vi "surface analysis.vi"() -> ()   [LabVIEW 2018]
uses:
  Program Files (x86)/National Instruments/LabVIEW 2018/examples/Connectivity/Python/support/PythonVersionsEnum.ctl
  PythonConfigGlobal.vi
panel:
  in  "탭 컨트롤":T1(tab)
  in  "python version":T2=enum."3.6"
  in  "auto select":bool=TRUE
  in  "p value 기준":dbl=0.30000000000000004 format="%#_13g"
  in  "min max":dbl[][](array[numeric])=[[4.0, 10.0], [50.0, 150.0], [0.5, 1.5]]
  in  "요인":string[](array[string])=["x1", "x2", "x3"]
  in  "비용목표":string[](array[string])=["y1"]
  in  "min":dbl[](array[numeric])
  in  "max":dbl[](array[numeric])
  out "최소화":bool[](array[boolean])
  out "CCD":dbl[][](array[numeric])=[[0.0, 1.0, 1.0], [-1.0, 0.0, -1.0], [1.0, -1.0, 0.0], [0.0, -1.0, 1.0], [0.0, 1.0, -1.0], [1.0, 1.0, 0.0], [0.0, 0.0, 0.0], [1.0, 0.0, 1.0], [0.0, 0.0, 0.0], [-1.0, -1.0, 0.0], [0.0, 0.0, 0.0], [-1.0, 0.0, 1.0], [1.0, 0.0, -1.0], [-1.0, 1.0, 0.0], [0.0, -1.0, -1.0]]
  out "요인 인디케이터":string[](array[string])=["x1", "x2", "x3"]
  out "결과":dbl[][](array[numeric])=[[-7664.4331863081525], [-4981.045086062967], [-2202.4239328817716], [-2350.3061672537383], [-7545.941821358417], [-7491.916698113938], [-4936.328310660356], [-4903.296353902461], [-4933.199416714428], [-2395.9779440706893], [-4933.81874642875], [-5116.35595558602], [-4793.002202085561], [-7680.887360331216], [-2246.212821164353]]
  out "비용 인디케이터":string[](array[string])=["y1"]
  out "시뮬레이션 인디케이터":string="시뮬레이션 횟수15/15\r\n인자 1 : 7.000000\r\n인자 2 : 50.000000\r\n인자 3 : 0.500000\r\n"
  in  "반복횟수":i32
  in  "정지":bool
  out "coef":dbl[](array[numeric])=[0.010139481576470908, 0.006600481306352523, 5.6726376890264e-10, 0.37234347257286826, 0.5641016129600653, 0.2140399578846797, 0.038152856088325596, 0.782518427242462, 0.17271126837436535, 0.40212171688452725]
  out "sumary":string="                            OLS Regression Results                            \n==============================================================================\nDep. Variable:                      y   R-squared:                       1.000\nModel:                            OLS   Adj. R-squared:                  1.000\nMethod:                 Least Squares   F-statistic:                 1.009e+05\nDate:                Sun, 20 Jan 2019   Prob (F-statistic):           1.32e-12\nTime:                        19:19:53   Log-Likelihood:                -43.985\nNo. Observations:                  15   AIC:                             108.0\nDf Residuals:                       5   BIC:                             115.0\nDf Model:                           9                                         \nCovariance Type:            nonrobust                                         \n==============================================================================\n                 coef    std err          t      P>|t|      [0.025      0.975]\n------------------------------------------------------------------------------\nconst        177.6892     44.222      4.018      0.010      64.013     291.365\nx1            33.1765      7.428      4.467      0.007      14.083      52.270\nx2           -52.3071      0.411   -127.305      0.000     -53.363     -51.251\nx3           -40.2432     41.088     -0.979      0.372    -145.863      65.377\nx4            -0.2808      0.455     -0.617      0.564      -1.450       0.889\nx5            -0.0023      0.002     -1.423      0.214      -0.007       0.002\nx6           -45.7962     16.377     -2.796      0.038     -87.893      -3.699\nx7            -0.0076      0.026     -0.291      0.783      -0.075       0.060\nx8             4.1695      2.622      1.590      0.173      -2.571      10.910\nx9            -0.1440      0.157     -0.915      0.402      -0.548       0.260\n==============================================================================\nOmnibus:                        0.092   Durbin-Watson:                   2.815\nProb(Omnibus):                  0.955   Jarque-Bera (JB):                0.320\nSkew:                          -0.003   Prob(JB):                        0.852\nKurtosis:                       2.284   Cond. No.                     3.73e+05\n==============================================================================\n\nWarnings:\n[1] Standard Errors assume that the covariance matrix of the errors is correctly specified.\n[2] The condition number is large, 3.73e+05. This might indicate that there are\nstrong multicollinearity or other numerical problems."
  out "name sort":string[](array[string])=["const", "x1 : x1", "x2 : x2", "x3 : x3", "x4 : x1^2", "x5 : x2^2", "x6 : x3^2", "x7 : x1*x2", "x8 : x1*x3", "x9 : x2*x3"]
  out "pValue sort":dbl[](array[numeric])=[0.010139481576470908, 0.006600481306352523, 5.6726376890264e-10, 0.37234347257286826, 0.5641016129600653, 0.2140399578846797, 0.038152856088325596, 0.782518427242462, 0.17271126837436535, 0.40212171688452725]
  in  "select":bool[](array[boolean])=[TRUE, TRUE, TRUE, TRUE, TRUE, TRUE, FALSE, FALSE, FALSE, FALSE]
  in  "선택완료":bool
  # "AUTO\nSELECT"
  # "1 2 3"
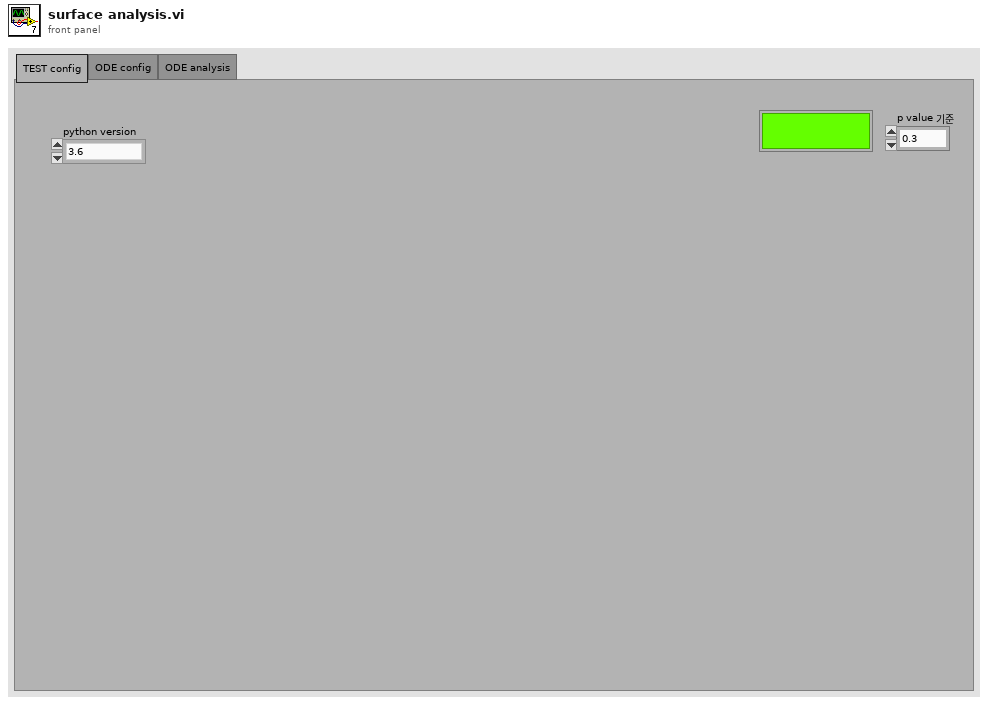
[diagram p1: front panel]
types:
  T1 = enum32{"TEST config", "ODE config", "ODE analysis"}
  T2 = typedef "PythonVersionsEnum.ctl" = enum16{"2.7", "3.6"}
  T3 = cluster{"session out":refnum<k35>, "appended path":path}
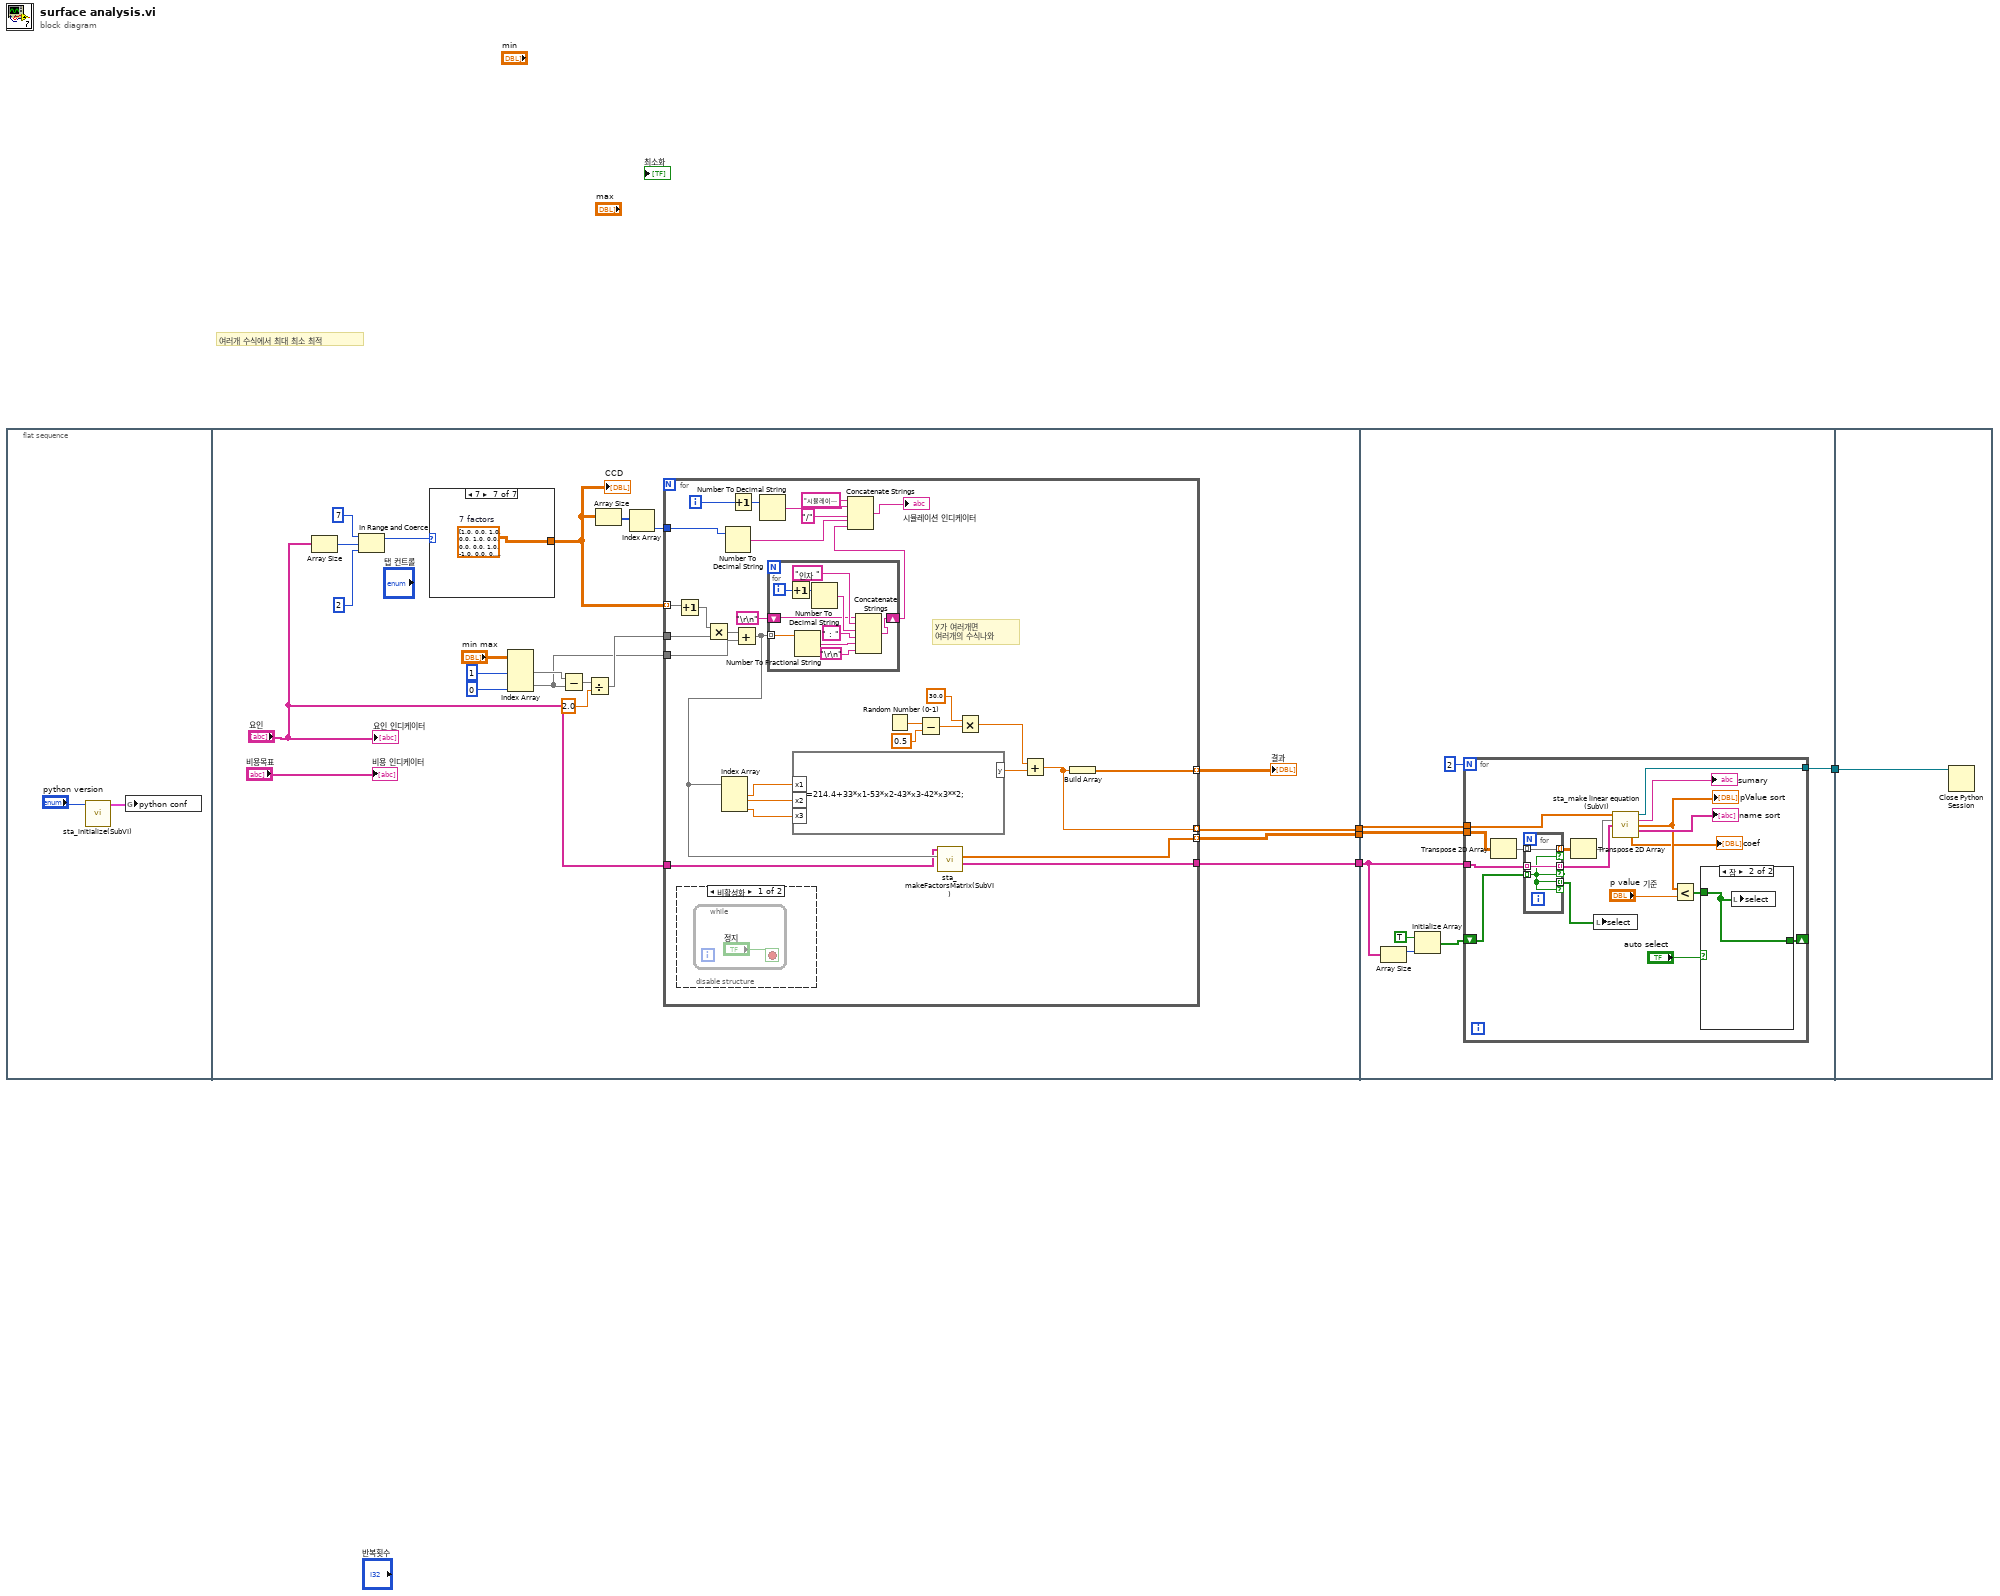
[diagram p0: block diagram]
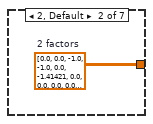
[diagram p4: hidden frame]
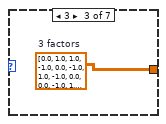
[diagram p5: hidden frame]
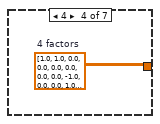
[diagram p6: hidden frame]
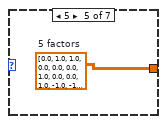
[diagram p7: hidden frame]
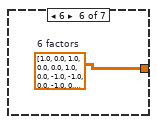
[diagram p8: hidden frame]
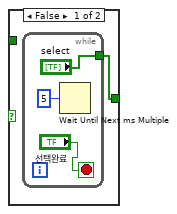
[diagram p9: hidden frame]
diagram:
  # "여러개 수식에서 최대 최소 최적"
  n1 = flat-sequence {
    tunnel: [w10] -> w4
    tunnel: [w9] -> w3
    tunnel: [w7] -> w1
    tunnel: w4 -> [w81]
    tunnel: w3 -> [w82]
    tunnel: [w80] -> w2
    tunnel: w1 -> [w77]
    tunnel: w2 -> [w109]
    frame #0 {
      n2 = call "sta_initialize(SubVI).vi"("python version"="python version") -> ("클러스터"=w5:T3)  [unwired: 10 in]
      n3 = global write "PythonConfigGlobal.vi" "python conf"(w5) -> ()
    }
    frame #1 {
      n4 = Array Size(array="요인") -> (size(s)=w26:i32)
      n5 = In Range and Coerce(upper limit=7 ("상위 리미트"), x=w26, lower limit=2 ("하위 리미트")) -> (coerced(x)=w23:i32)  [unwired: 1 out]
      n6 = case shown="7" w23 {
        tunnel: [_ w69 w70 w71 w72 w73 w74] -> w22
        frame 1 {
          # "황금비 추가"
        }
        frame 2, Default {
          w69 = dbl[][] [[0.0, 0.0], [-1.0, -1.0], [0.0, -1.41421], [0.0, 0.0], [0.0, 0.0], [1.41421, 0.0], [-1.0, 1.0], [-1.41421, 0.0], [0.0, 1.41421], [1.0, 1.0], [1.0, -1.0], [0.0, 0.0], [0.0, 0.0]]  # 2 factors
        }
        frame 3 {
          w70 = dbl[][] [[0.0, 1.0, 1.0], [-1.0, 0.0, -1.0], [1.0, -1.0, 0.0], [0.0, -1.0, 1.0], [0.0, 1.0, -1.0], [1.0, 1.0, 0.0], [0.0, 0.0, 0.0], [1.0, 0.0, 1.0], [0.0, 0.0, 0.0], [-1.0, -1.0, 0.0], [0.0, 0.0, 0.0], [-1.0, 0.0, 1.0], [1.0, 0.0, -1.0], [-1.0, 1.0, 0.0], [0.0, -1.0, -1.0]]  # 3 factors
        }
        frame 4 {
          w71 = dbl[][] [[1.0, 1.0, 0.0, 0.0], [0.0, 0.0, 0.0, 0.0], [-1.0, 0.0, 0.0, 1.0], [-1.0, -1.0, 0.0, 0.0], [0.0, 1.0, 1.0, 0.0], [-1.0, 0.0, 0.0, -1.0], [0.0, 0.0, 1.0, 1.0], [0.0, -1.0, -1.0, 0.0], [1.0, 0.0, -1.0, 0.0], [0.0, -1.0, 1.0, 0.0], [1.0, -1.0, 0.0, 0.0], [0.0, -1.0, 0.0, 1.0], [-1.0, 0.0, -1.0, 0.0], [0.0, 0.0, 0.0, 0.0], [1.0, 0.0, 0.0, -1.0], [1.0, 0.0, 0.0, 1.0], [0.0, -1.0, 0.0, -1.0], [0.0, 1.0, 0.0, 1.0], [0.0, 1.0, -1.0, 0.0], [-1.0, 0.0, 1.0, 0.0], [0.0, 0.0, 1.0, -1.0], [0.0, 0.0, -1.0, -1.0], [1.0, 0.0, 1.0, 0.0], [0.0, 0.0, 0.0, 0.0], [0.0, 1.0, 0.0, -1.0], [-1.0, 1.0, 0.0, 0.0], [0.0, 0.0, -1.0, 1.0]]  # 4 factors
        }
        frame 5 {
          w72 = dbl[][] [[0.0, 1.0, 1.0, 0.0, 0.0], [0.0, 1.0, 0.0, 0.0, 1.0], [-1.0, -1.0, 0.0, 0.0, 0.0], [0.0, 1.0, -1.0, 0.0, 0.0], [0.0, 0.0, 0.0, 0.0, 0.0], [0.0, 0.0, 0.0, 1.0, 1.0], [1.0, 1.0, 0.0, 0.0, 0.0], [0.0, 1.0, 0.0, 1.0, 0.0], [-1.0, 0.0, 1.0, 0.0, 0.0], [1.0, 0.0, 0.0, -1.0, 0.0], [0.0, 1.0, 0.0, 0.0, -1.0], [0.0, 0.0, 1.0, -1.0, 0.0], [0.0, 0.0, 0.0, 0.0, 0.0], [-1.0, 0.0, 0.0, -1.0, 0.0], [-1.0, 0.0, 0.0, 1.0, 0.0], [0.0, -1.0, 0.0, 1.0, 0.0], [0.0, 1.0, 0.0, -1.0, 0.0], [-1.0, 0.0, 0.0, 0.0, -1.0], [0.0, 0.0, 1.0, 0.0, -1.0], [0.0, 0.0, 0.0, 0.0, 0.0], [1.0, 0.0, 0.0, 0.0, 1.0], [1.0, -1.0, 0.0, 0.0, 0.0], [0.0, 0.0, 0.0, 1.0, -1.0], [0.0, 0.0, -1.0, 0.0, -1.0], [-1.0, 1.0, 0.0, 0.0, 0.0], [0.0, 0.0, 0.0, 0.0, 0.0], [0.0, 0.0, -1.0, -1.0, 0.0], [1.0, 0.0, -1.0, 0.0, 0.0], [0.0, 0.0, 1.0, 0.0, 1.0], [0.0, -1.0, 1.0, 0.0, 0.0], [0.0, -1.0, -1.0, 0.0, 0.0], [1.0, 0.0, 0.0, 0.0, -1.0], [1.0, 0.0, 1.0, 0.0, 0.0], [0.0, -1.0, 0.0, 0.0, -1.0], [-1.0, 0.0, 0.0, 0.0, 1.0], [0.0, -1.0, 0.0, 0.0, 1.0], [0.0, 0.0, 0.0, -1.0, 1.0], [0.0, -1.0, 0.0, -1.0, 0.0], [0.0, 0.0, -1.0, 1.0, 0.0], [1.0, 0.0, 0.0, 1.0, 0.0], [0.0, 0.0, 0.0, -1.0, -1.0], [-1.0, 0.0, -1.0, 0.0, 0.0], [0.0, 0.0, 1.0, 1.0, 0.0], [0.0, 0.0, 0.0, 0.0, 0.0], [0.0, 0.0, 0.0, 0.0, 0.0], [0.0, 0.0, -1.0, 0.0, 1.0]]  # 5 factors
        }
        frame 6 {
          w73 = dbl[][] [[1.0, 0.0, 1.0, 0.0, 0.0, 1.0], [0.0, -1.0, -1.0, 0.0, -1.0, 0.0], [-1.0, 0.0, -1.0, 0.0, 0.0, -1.0], [-1.0, 0.0, 0.0, 1.0, 1.0, 0.0], [-1.0, 1.0, 0.0, 1.0, 0.0, 0.0], [1.0, 0.0, 0.0, -1.0, 1.0, 0.0], [-1.0, 0.0, -1.0, 0.0, 0.0, 1.0], [-1.0, 0.0, 1.0, 0.0, 0.0, -1.0], [0.0, -1.0, 0.0, 0.0, 1.0, 1.0], [1.0, 0.0, 0.0, -1.0, -1.0, 0.0], [0.0, 1.0, 0.0, 0.0, 1.0, 1.0], [0.0, 1.0, 0.0, 0.0, 1.0, -1.0], [1.0, -1.0, 0.0, -1.0, 0.0, 0.0], [1.0, 1.0, 0.0, 1.0, 0.0, 0.0], [1.0, 0.0, -1.0, 0.0, 0.0, -1.0], [0.0, 0.0, -1.0, -1.0, 0.0, -1.0], [0.0, 1.0, 1.0, 0.0, -1.0, 0.0], [-1.0, 0.0, 0.0, 1.0, -1.0, 0.0], [0.0, 0.0, 0.0, 0.0, 0.0, 0.0], [-1.0, 0.0, 0.0, -1.0, 1.0, 0.0], [0.0, 1.0, -1.0, 0.0, -1.0, 0.0], [0.0, -1.0, 0.0, 0.0, -1.0, 1.0], [0.0, 1.0, 0.0, 0.0, -1.0, 1.0], [-1.0, 0.0, 1.0, 0.0, 0.0, 1.0], [0.0, 0.0, 0.0, 0.0, 0.0, 0.0], [0.0, 0.0, 0.0, 0.0, 0.0, 0.0], [-1.0, 0.0, 0.0, -1.0, -1.0, 0.0], [0.0, 0.0, 1.0, 1.0, 0.0, -1.0], [1.0, 0.0, 0.0, 1.0, -1.0, 0.0], [0.0, 0.0, 0.0, 0.0, 0.0, 0.0], [-1.0, 1.0, 0.0, -1.0, 0.0, 0.0], [0.0, 1.0, 0.0, 0.0, -1.0, -1.0], [0.0, -1.0, 1.0, 0.0, 1.0, 0.0], [1.0, 0.0, 0.0, 1.0, 1.0, 0.0], [-1.0, -1.0, 0.0, -1.0, 0.0, 0.0], [0.0, 0.0, -1.0, 1.0, 0.0, -1.0], [0.0, 0.0, 1.0, -1.0, 0.0, 1.0], [0.0, 1.0, 1.0, 0.0, 1.0, 0.0], [-1.0, -1.0, 0.0, 1.0, 0.0, 0.0], [0.0, 0.0, -1.0, 1.0, 0.0, 1.0], [0.0, 0.0, 0.0, 0.0, 0.0, 0.0], [1.0, 1.0, 0.0, -1.0, 0.0, 0.0], [0.0, 0.0, -1.0, -1.0, 0.0, 1.0], [0.0, 0.0, 1.0, -1.0, 0.0, -1.0], [1.0, -1.0, 0.0, 1.0, 0.0, 0.0], [0.0, 0.0, 1.0, 1.0, 0.0, 1.0], [0.0, 1.0, -1.0, 0.0, 1.0, 0.0], [0.0, -1.0, 0.0, 0.0, -1.0, -1.0], [1.0, 0.0, -1.0, 0.0, 0.0, 1.0], [0.0, -1.0, 0.0, 0.0, 1.0, -1.0], [0.0, -1.0, -1.0, 0.0, 1.0, 0.0], [0.0, 0.0, 0.0, 0.0, 0.0, 0.0], [0.0, -1.0, 1.0, 0.0, -1.0, 0.0], [1.0, 0.0, 1.0, 0.0, 0.0, -1.0]]  # 6 factors
        }
        frame 7 {
          w74 = dbl[][] [[1.0, 0.0, 1.0, 0.0, 1.0, 0.0, 0.0], [0.0, 1.0, -1.0, 0.0, 0.0, 1.0, 0.0], [-1.0, 0.0, 0.0, 0.0, 0.0, -1.0, 1.0], [0.0, 0.0, 1.0, 1.0, 0.0, 0.0, 1.0], [1.0, -1.0, 0.0, 1.0, 0.0, 0.0, 0.0], [0.0, 0.0, 0.0, 0.0, 0.0, 0.0, 0.0], [1.0, -1.0, 0.0, -1.0, 0.0, 0.0, 0.0], [0.0, 0.0, -1.0, -1.0, 0.0, 0.0, 1.0], [0.0, 0.0, 0.0, 0.0, 0.0, 0.0, 0.0], [1.0, 0.0, 0.0, 0.0, 0.0, 1.0, 1.0], [0.0, 1.0, 0.0, 0.0, 1.0, 0.0, -1.0], [0.0, 0.0, 1.0, -1.0, 0.0, 0.0, 1.0], [-1.0, 0.0, -1.0, 0.0, -1.0, 0.0, 0.0], [0.0, -1.0, 0.0, 0.0, 1.0, 0.0, -1.0], [0.0, 0.0, -1.0, 1.0, 0.0, 0.0, -1.0], [0.0, -1.0, -1.0, 0.0, 0.0, 1.0, 0.0], [1.0, 0.0, 0.0, 0.0, 0.0, -1.0, -1.0], [1.0, 1.0, 0.0, -1.0, 0.0, 0.0, 0.0], [0.0, 1.0, 1.0, 0.0, 0.0, 1.0, 0.0], [0.0, 0.0, 0.0, -1.0, -1.0, 1.0, 0.0], [0.0, 1.0, 0.0, 0.0, 1.0, 0.0, 1.0], [0.0, 0.0, 0.0, 1.0, 1.0, -1.0, 0.0], [0.0, -1.0, 1.0, 0.0, 0.0, 1.0, 0.0], [-1.0, -1.0, 0.0, -1.0, 0.0, 0.0, 0.0], [1.0, 0.0, 0.0, 0.0, 0.0, -1.0, 1.0], [0.0, 1.0, -1.0, 0.0, 0.0, -1.0, 0.0], [0.0, 0.0, -1.0, -1.0, 0.0, 0.0, -1.0], [0.0, -1.0, 1.0, 0.0, 0.0, -1.0, 0.0], [0.0, -1.0, -1.0, 0.0, 0.0, -1.0, 0.0], [-1.0, 1.0, 0.0, -1.0, 0.0, 0.0, 0.0], [-1.0, 1.0, 0.0, 1.0, 0.0, 0.0, 0.0], [1.0, 1.0, 0.0, 1.0, 0.0, 0.0, 0.0], [0.0, 0.0, 0.0, 1.0, -1.0, 1.0, 0.0], [0.0, 0.0, 0.0, -1.0, 1.0, 1.0, 0.0], [0.0, 0.0, 0.0, -1.0, -1.0, -1.0, 0.0], [0.0, 1.0, 0.0, 0.0, -1.0, 0.0, -1.0], [0.0, 0.0, 1.0, -1.0, 0.0, 0.0, -1.0], [-1.0, 0.0, 1.0, 0.0, -1.0, 0.0, 0.0], [0.0, 0.0, 0.0, -1.0, 1.0, -1.0, 0.0], [-1.0, -1.0, 0.0, 1.0, 0.0, 0.0, 0.0], [0.0, 0.0, 0.0, 0.0, 0.0, 0.0, 0.0], [-1.0, 0.0, -1.0, 0.0, 1.0, 0.0, 0.0], [1.0, 0.0, -1.0, 0.0, 1.0, 0.0, 0.0], [0.0, 1.0, 1.0, 0.0, 0.0, -1.0, 0.0], [0.0, 0.0, 0.0, 0.0, 0.0, 0.0, 0.0], [0.0, 0.0, 0.0, 1.0, 1.0, 1.0, 0.0], [0.0, 1.0, 0.0, 0.0, -1.0, 0.0, 1.0], [0.0, 0.0, 0.0, 1.0, -1.0, -1.0, 0.0], [-1.0, 0.0, 1.0, 0.0, 1.0, 0.0, 0.0], [0.0, 0.0, 0.0, 0.0, 0.0, 0.0, 0.0], [0.0, 0.0, -1.0, 1.0, 0.0, 0.0, 1.0], [0.0, -1.0, 0.0, 0.0, -1.0, 0.0, -1.0], [0.0, 0.0, 0.0, 0.0, 0.0, 0.0, 0.0], [-1.0, 0.0, 0.0, 0.0, 0.0, 1.0, 1.0], [1.0, 0.0, 1.0, 0.0, -1.0, 0.0, 0.0], [-1.0, 0.0, 0.0, 0.0, 0.0, 1.0, -1.0], [1.0, 0.0, -1.0, 0.0, -1.0, 0.0, 0.0], [0.0, 0.0, 1.0, 1.0, 0.0, 0.0, -1.0], [-1.0, 0.0, 0.0, 0.0, 0.0, -1.0, -1.0], [0.0, -1.0, 0.0, 0.0, 1.0, 0.0, 1.0], [1.0, 0.0, 0.0, 0.0, 0.0, 1.0, -1.0], [0.0, -1.0, 0.0, 0.0, -1.0, 0.0, 1.0]]  # 7 factors
        }
      }
      "CCD" <- w22
      n7 = Index Array(array="min max", index (col) #1=1 ("비활성화된 인덱스 (열)"), index (col) #2=0 ("인덱스 (열)")) -> (element #1=w13:dbl[], element #2=w12:dbl[])  [unwired: 2 in]
      n8 = Subtract(x=w13, y=w12) -> (x-y=w16:dbl[])
      n9 = Divide(x=w16, y=2.0) -> (x/y=w14:dbl[])
      n10 = Array Size(array=w22) -> (size(s)=w21:i32[])
      n11 = Index Array(array=w21) -> (element=w20:i32)  [unwired: 1 in]
      n12 = for {
        tunnel: w22 -> [w47] mode=indexing
        tunnel: w20 -> [w53]
        tunnel: w14 -> [w46]
        tunnel: w12 -> [w45]
        tunnel: [w42] -> w11 mode=indexing
        tunnel: [w38] -> w10 mode=indexing
        tunnel: [w31] -> w9 mode=indexing
        tunnel: "요인" -> [w29]
        tunnel: [w28] -> w7
        i -> [w51]
        # "y가 여러개면\n여러개의 수식나와"
        n13 = Increment(x=w47) -> (x+1=w48:dbl[])
        n14 = disable-structure shown="비활성화" {
          frame Disabled {
            n15 = while {
              stop <- "정지" stop-if-true
            }
          }
          frame Enabled {
          }
        }
        n16 = Multiply(x=w48, y=w46) -> (x*y=w49:dbl[])
        n17 = Number To Decimal String(number=w53) -> (decimal integer string=w52:string)  [unwired: 1 in]
        n18 = Increment(x=w51) -> (x+1=w50:i32)
        n19 = Add(x=w49, y=w45) -> (x+y=w30:dbl[])
        n20 = Index Array(array=w30) -> (element #1=w41:dbl, element #2=w40:dbl, element #3=w39:dbl)  [unwired: 3 in]
        n21 = Number To Decimal String(number=w50) -> (decimal integer string=w56:string)  [unwired: 1 in]
        n22 = for {
          tunnel: w30 -> [w63] mode=indexing
          shift-right: [w60] -> w43
          shift-left: "\r\n" -> [w61]
          i -> [w67]
          n23 = Increment(x=w67) -> (x+1=w68:i32)
          n24 = Number To Fractional String(number=w63) -> (F-format string=w62:string)  [unwired: 3 in]
          n25 = Number To Decimal String(number=w68) -> (decimal integer string=w66:string)  [unwired: 1 in]
          n26 = Concatenate Strings(w61, "인자 " ("문자열"), w66, " : " ("문자열"), w62, "\r\n") -> (w60:string)
        }
        n27 = formula code="y=214.4+33*x1-53*x2-43*x3-42*x3**2;"("x1"=w41, "x2"=w40, "x3"=w39) -> ("y"=w33:dbl)
        n28 = Concatenate Strings("시뮬레이션 횟수" ("문자열"), w56, "/" ("문자열"), w52, w43) -> (→"시뮬레이션 인디케이터":string)
        n29 = Random Number (0-1)() -> (number: 0 to 1=w37:dbl)
        n30 = Subtract(x=w37, y=0.5) -> (x-y=w35:dbl)
        n31 = call "sta_makeFactorsMatrix(SubVI).vi"("factors 입력"=w30, "factors name"=w29) -> ("name"=w28:string[], "factors 출력"=w38:dbl[])  [unwired: 6 in, 2 out]
        n32 = Multiply(x=30.0, y=w35) -> (x*y=w32:dbl)
        n33 = Add(x=w32, y=w33) -> (x+y=w31:dbl)
        n34 = Build Array(w31) -> (w42:dbl[])
      }
      "결과" <- w11
      "요인 인디케이터" <- "요인"
      "비용 인디케이터" <- "비용목표"
    }
    frame #2 {
      n35 = Array Size(array=w77) -> (size(s)=w76:i32)
      n36 = Initialize Array(TRUE, w76) -> (w75:bool[])
      n37 = for {
        N: 2 -> [_]
        tunnel: w82 -> [w98]
        tunnel: w81 -> [w90]
        tunnel: [w97] -> w80
        tunnel: w77 -> [w91]
        shift-right: [w92] -> _
        shift-left: w75 -> [w85]
        n38 = Transpose 2D Array(2D array=w90) -> (transposed array=w89:dbl[][])
        n39 = for {
          tunnel: w85 -> [w101] mode=indexing
          tunnel: w91 -> [w102] mode=indexing
          tunnel: w89 -> [w103] mode=indexing
          tunnel: [w103] -> w88 mode=indexing if=w101
          tunnel: [w102] -> w86 mode=indexing if=w101
          tunnel: [w101] -> w84 mode=indexing if=w101
        }
        n40 = Transpose 2D Array(2D array=w88) -> (transposed array=w87:dbl[][])
        n41 = local write "select"(w84) -> ()
        n42 = call "sta_make linear equation (SubVI).vi"("test result"=w98, "factors"=w87, "name"=w86) -> ("참조 번호 출력"=w97:refnum<k35>, "sumary"=→"sumary":string, "pValue sort"=w96:dbl[], "name sort"=→"name sort":string[], "coef"=→"coef":dbl[])  [unwired: 7 in, 1 out]
        "pValue sort" <- w96
        n43 = Less?(x=w96, y="p value 기준") -> (x < y?=w94:bool[])
        n44 = case shown="참" "auto select" {
          tunnel: w94 -> [_ w108]
          tunnel: [w104 w108] -> w92
          frame False {
            n45 = while {
              tunnel: ["select"] -> w104
              stop <- "선택완료" stop-if-true
              n46 = Wait Until Next ms Multiple(millisecond multiple=u32 5 ("ms 배수")) -> ()  [unwired: 1 out]
            }
          }
          frame True {
            n47 = local write "select"(w108) -> ()
          }
        }
      }
    }
    frame #3 {
      n48 = Close Python Session(session in=w109) -> ()  [unwired: 1 in, 1 out]
    }
  }
